vi "LogAndClearError.vi"(7 "Log and view ?":T2, 8 "error in (no error)":errorcluster, 9 "type of dialog":T1 items=["no dialog", "OK message", "continue or stop message", "OK message + warnings", "continue/stop + warnings"]) -> (0 "error out":errorcluster)   [LabVIEW 2013]
uses:
  Ctrls/enumLogAndView.ctl
  <vilib>/Utility/error.llb/DialogType.ctl
  030 - EVENTS/03 - ToMessageHandlerProcess/ToMessageHandlerEvent.ctl
  030 - EVENTS/03 - ToMessageHandlerProcess/enumMessageCriticity.ctl
  030 - EVENTS/EnumFgvEventCommand.ctl
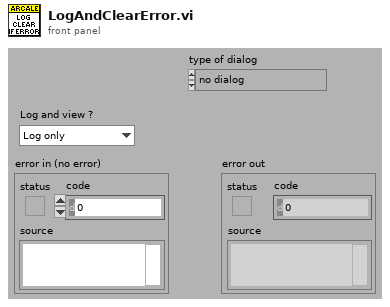
[diagram p1: front panel]
types:
  T1 = typedef "DialogType.ctl" = u16
  T2 = typedef "enumLogAndView.ctl" = enum16{"Log only", "Log and view"}
  T3 = typedef "enumMessageCriticity.ctl" = enum16{"No error", "Info", "Warning", "Error", "Fatal error"}
  T4 = typedef "ToMessageHandlerEvent.ctl" = cluster{"date / time":timestamp, "Criticity":T3, "Emitter":string, "Message":string}
  T5 = typedef "EnumFgvEventCommand.ctl" = enum16{"Setup", "Cleanup", "Get"}
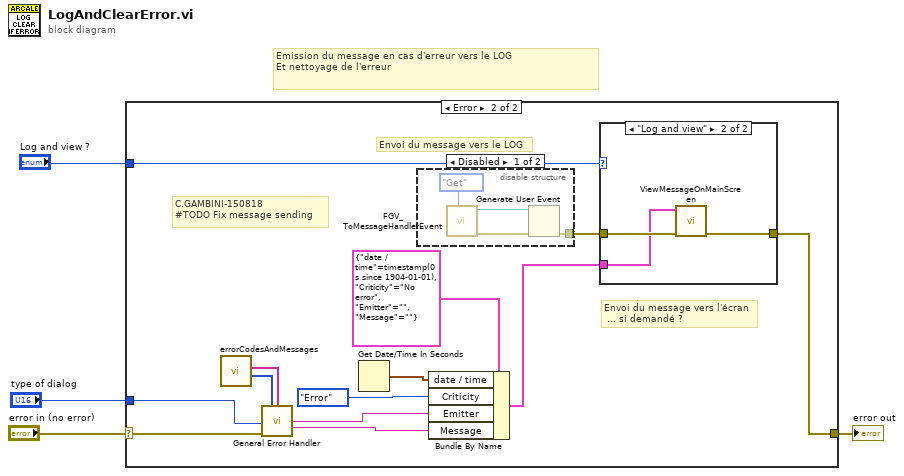
[diagram p0: block diagram]
diagram:
  # "Emission du message en cas d'erreur vers le LOG\nEt nettoyage de l'erreur"
  n1 = case shown="Error" "error in (no error)" {
    selector: "error in (no error)" -> [w5 w16]
    tunnel: [w5 w8] -> w3
    tunnel: "Log and view ?" -> [_ w10]
    tunnel: "type of dialog" -> [_ w6]
    frame No Error {
    }
    frame Error {
      # "C.GAMBINI-150818\n#TODO Fix message sending"
      # "Envoi du message vers l'écran\n ... si demandé ?"
      # "Envoi du message vers le LOG"
      n2 = call "errorCodesAndMessages.vi"() -> ("errorCodes"=w18:i32[], "errorMessages"=w17:string[])  [unwired: 10 out]
      n3 = call <vilib>:"General Error Handler.vi"("[user-defined codes]"=w18, "[user-defined descriptions]"=w17, "type of dialog (OK msg:1)"=w6, "error in (no error)"=w16) -> ("source out"=w12:string, "message"=w11:string)  [unwired: 10 out]
      n4 = Get Date/Time In Seconds() -> (seconds since 1Jan1904=w14:timestamp)
      n5 = disable-structure shown="Disabled" {
        disable-tunnel: [w19 _] -> w9
        frame Disabled {
          n6 = call "FGV_ToMessageHandlerEvent.vi"("Command"=EnumFgvEventCommand."Get") -> ("error out"=w21:errorcluster, "To message handler event"=w20:refnum<user-event>)  [unwired: 9 in]
          n7 = Generate User Event(user event=w20, error in=w21) -> (error out=w19:errorcluster)  [unwired: 2 in, 1 out]
        }
        frame Enabled {
        }
      }
      n8 = Bundle By Name(cluster=T4 {"date / time"=timestamp(0 s since 1904-01-01), "Criticity"=enum."No error", "Emitter"="", "Message"=""} ("event data"), "date / time"=w14, "Criticity"=enumMessageCriticity."Error", "Emitter"=w12, "Message"=w11) -> (w7:T4)
      n9 = case shown="\"Log and view\"" w10 {
        tunnel: w9 -> [w23 w26]
        tunnel: [w23 w25] -> w8
        tunnel: w7 -> [_ w24]
        frame "Log only" {
        }
        frame "Log and view" {
          n10 = call "ViewMessageOnMainScreen.vi"("error in (no error)"=w26, "Message"=w24) -> ("error out"=w25:errorcluster)  [unwired: 9 in]
        }
      }
    }
  }
  "error out" <- w3
